vi "start_operation.vi"() -> ()   [LabVIEW 2017]
uses:
  controls/DisplayCommanda.ctl
  DisplayControl-czyjes.ctl
  controls/EnableDisableCmd.ctl
  Downloads/ATM Simulator/Controls/DisplayCommand.ctl
  Downloads/ATM Simulator/Controls/DisplayControl.ctl
panel:
  in  "queue":refnum<queue>
  out "queue out":refnum<queue>
  out "error out":errorcluster
  in  "error in (no error)":errorcluster
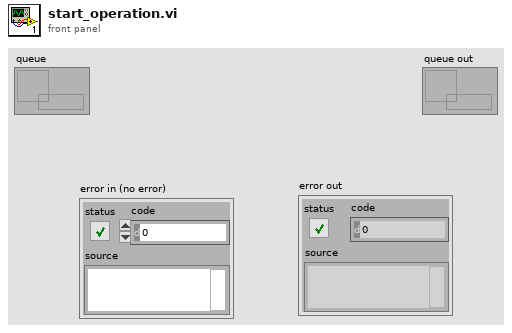
[diagram p1: front panel]
types:
  T1 = typedef "DisplayControl-czyjes.ctl" = cluster{"Command":T2, "Data":variant}
  T2 = typedef "DisplayCommanda.ctl" = enum16{"Initialize", "StartOperation", "Enable/Disable Controls", "FocusCursor", "UpdateMessage", "UpdateMenus", "FinishOperation", "Exit", "CleanUserInput"}
  T3 = typedef "EnableDisableCmd.ctl" = enum16{"InitialSetup", "Disable Menus", "Enable Menus", "Disable User Input", "Enable User Input"}
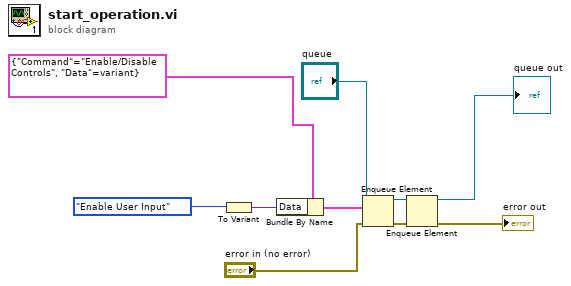
[diagram p0: block diagram]
diagram:
  n1 = To Variant(anything=EnableDisableCmd."Enable User Input" ("Enable/Disable Command")) -> (Variant=w9:variant)
  n2 = Bundle By Name(cluster=T1 {"Command"=enum."Enable/Disable Controls", "Data"=variant} ("DisplayControl"), "Data"=w9) -> (w1:T1)
  n3 = Enqueue Element(queue="queue", element=w1, error in (no error)="error in (no error)") -> (queue out=w5:refnum<queue>, error out=w8:errorcluster)  [unwired: 1 in, 1 out]
  n4 = Enqueue Element(queue=w5, error in (no error)=w8) -> (queue out=→"queue out":refnum<queue>, error out=→"error out":errorcluster)  [unwired: 2 in, 1 out]
